vi "Read.vi"() -> ()   [LabVIEW 2023]
uses:
  <vilib>/OPCUA/client/Multiple Read Double.vi
  <vilib>/OPCUA/NI OPC UA Client.lvlib
panel:
  in  "Stop Button":bool
  in  "Item Path":string="ns=2;s=Tag1"
  in  "Server Endpoint URL":string="opc.tcp://beist:62640/IntegrationObjects/ServerSimulator"
  out "Read Number":dbl
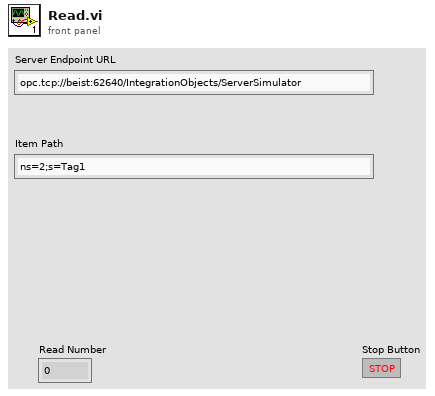
[diagram p1: front panel]
types:
  T1 = cluster{"message mode":enum16{"None", "Sign", "Sign and Encrypt"}, "security":enum16{"Basic256", "Basic128Rsa15"}}
  T2 = typedef "OPC UA Client Refnum.ctl" = refnum<k21>
  T3 = typedef "NodeId.ctl" = string
  T4 = typedef "OPC UA StatusCode.ctl" = u32
  T5 = cluster{"node ID":T3, "value ":dbl, "timestamp":timestamp, "status":T4}[]
  T6 = cluster{"node ID":T3, "value ":dbl, "timestamp":timestamp, "status":T4}
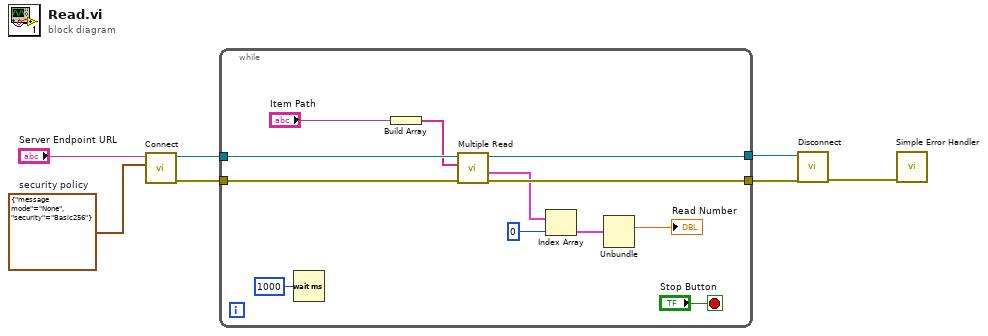
[diagram p0: block diagram]
diagram:
  w6 = T1 {"message mode"=enum."None", "security"=enum."Basic256"}  # security policy
  n1 = call <vilib>:"Connect.vi"("security policy"=w6, "server endpoint URL"="Server Endpoint URL") -> ("error out"=w3:errorcluster, "OPC UA client refnum out"=w5:T2)  [unwired: 7 in, 1 out]
  n2 = while {
    tunnel: w5 -> [w17]
    tunnel: [w16] -> w4
    tunnel: w3 -> [w15]
    tunnel: [w14] -> w2
    stop <- "Stop Button" stop-if-true
    n3 = Wait (ms)(milliseconds to wait=u32 1000) -> ()  [unwired: 1 out]
    n4 = Build Array "Build Array"("Item Path") -> (w12:string[])
    n5 = call-poly <vilib>:"Multiple Read.vi"("error in (no error)"=w15, "node IDs"=w12, "OPC UA client refnum in"=w17) -> ("error out"=w14:errorcluster, "results"=w10:T5, "OPC UA client refnum out"=w16:T2)  [unwired: 5 in, 1 out]
    n6 = Index Array "Index Array"(array=w10, index=0) -> (element=w9:T6)
    n7 = Unbundle "Unbundle"(w9) -> ("value"=→"Read Number":dbl)  [unwired: 3 out]
  }
  n8 = call <vilib>:"Disconnect.vi"("error in (no error)"=w2, "OPC UA client refnum in"=w4) -> ("error out"=w1:errorcluster)  [unwired: 9 in]
  n9 = call <vilib>:"Simple Error Handler.vi"("error in (no error)"=w1) -> ()  [unwired: 4 in, 5 out]
